vi "Create Plot Object.vi"(6 "Control Ref Queue":T1, 7 "Actual Transform In":T2, 8 "error in (no error)":errorcluster, 9 "Multiplot Representation In":T4, 10 "3D Mesh.lvclass in":refnum<class "3D Waterfall.lvclass">, 11 "Plot Object In":refnum<vi>) -> (0 "error out":errorcluster, 1 "Multiplot Representation Out":T4, 2 "3D Mesh.lvclass out":refnum<class "3D Waterfall.lvclass">, 3 "Plot Object Out":refnum<vi>, 5 "Actual Transform Out":T2)   [LabVIEW 2017, in "3D Waterfall.lvclass"]
uses:
  <vilib>/Math Plots/3D Math Plots/3D Waterfall/3D Waterfall/3D Waterfall.lvclass
  <vilib>/Math Plots/3D Math Plots/3D Plot/3D Plot/Typedef/Multiplot Representation.ctl
  <vilib>/Math Plots/3D Math Plots/3D Plot/3D Plot/Typedef/Plot Representation.ctl
  <vilib>/Math Plots/3D Math Plots/3D Plot/3D Plot/Typedef/Range Clusters.ctl
  <vilib>/Math Plots/3D Math Plots/3D Plot/3D Plot/Typedef/Mesh Data.ctl
  <vilib>/Math Plots/3D Math Plots/3D Plot/3D Plot/Typedef/Actual Transform.ctl
  <vilib>/Math Plots/3D Math Plots/3D Plot/Action String/3DMathPlot Ctrl Act Queue.ctl
  <vilib>/Math Plots/3D Math Plots/3D Plot/Action String/3DMathPlot Ctrl Act Cluster.ctl
  <vilib>/Math Plots/3D Math Plots/3D Plot/Action String/3DMathPlot State Class.ctl
  <vilib>/Math Plots/3D Math Plots/3D Waterfall/3D Waterfall/3D Waterfall.lvclass/3D Waterfall.ctl
  <vilib>/Math Plots/3D Math Plots/3D Plot/3D Plot/3D Plot.lvclass
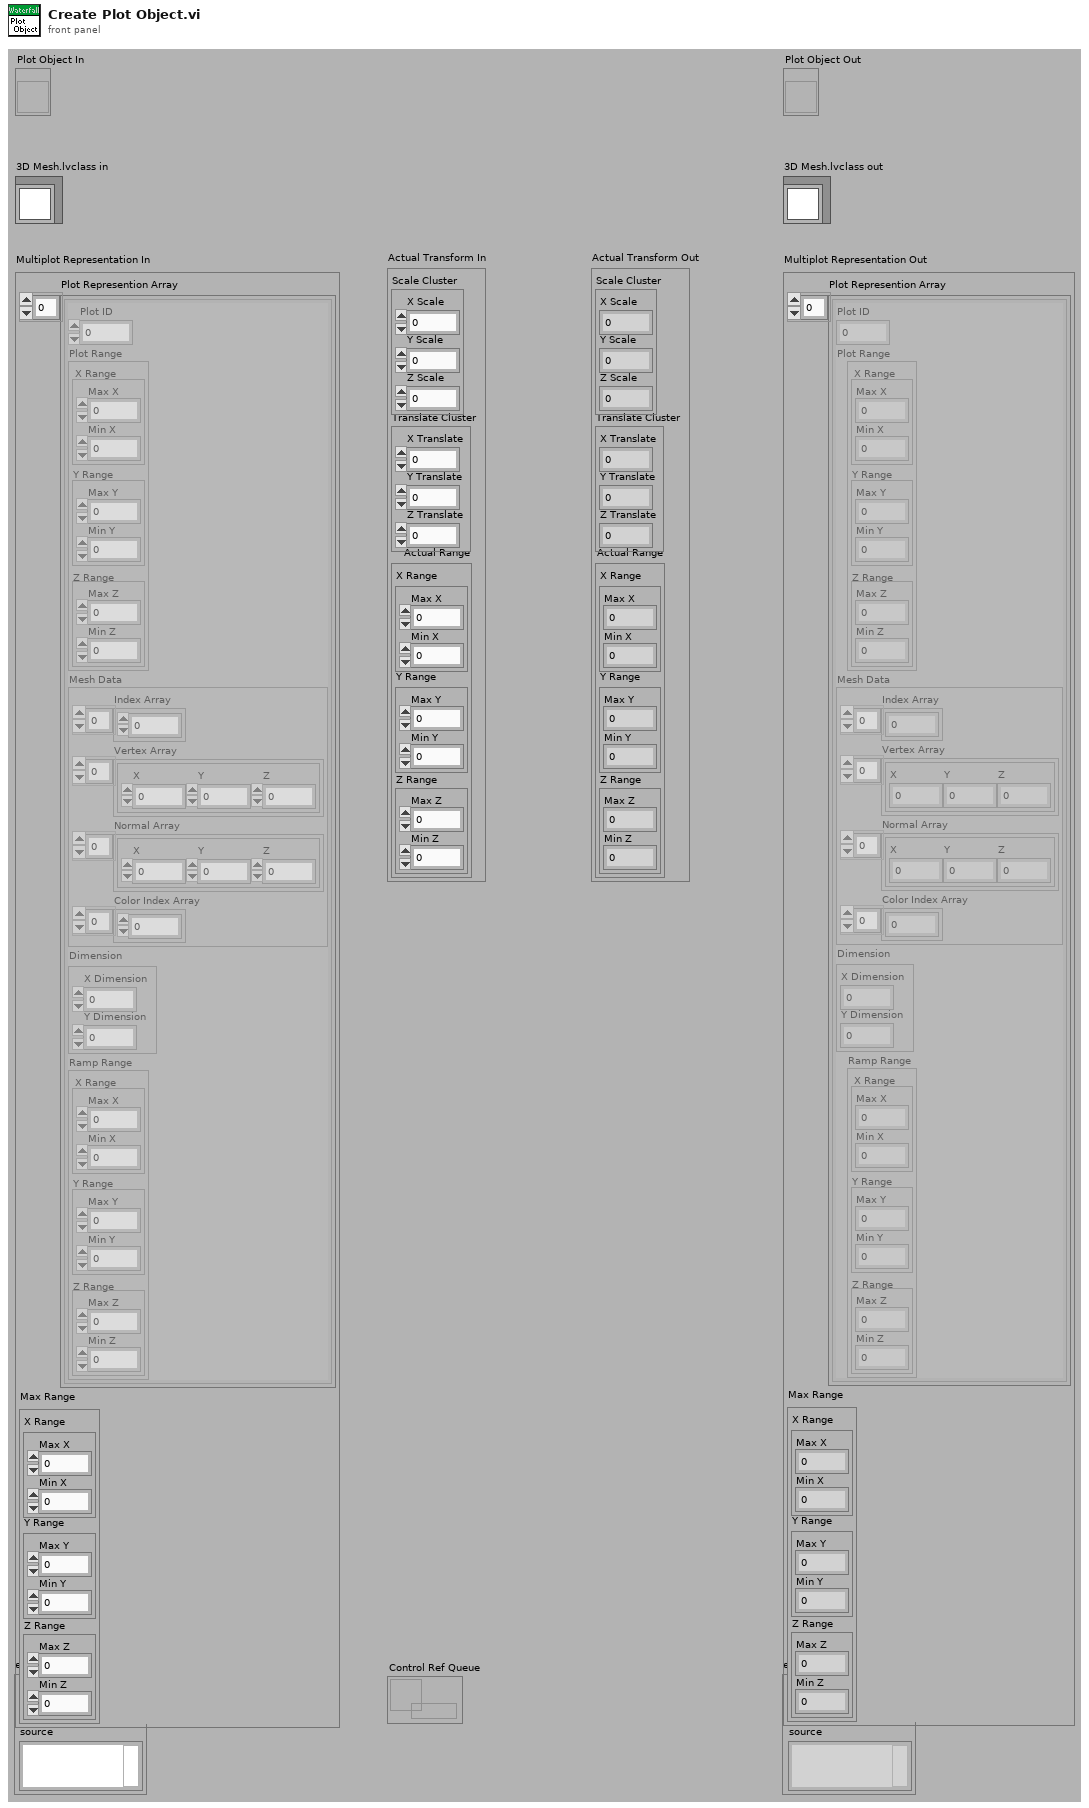
[diagram p1: front panel]
types:
  T1 = typedef "3DMathPlot Ctrl Act Queue.ctl" = refnum<queue>
  T2 = typedef "3D Plot.lvclass/Actual Transform.ctl" = cluster{"Scale Cluster":cluster{"X Scale":sgl, "Y Scale":sgl, "Z Scale":sgl}, "Translate Cluster":cluster{"X Translate":sgl, "Y Translate":sgl, "Z Translate":sgl}, "Actual Range":T3}
  T3 = typedef "3D Plot.lvclass/Range Clusters.ctl" = cluster{"X Range":cluster{"Max X":sgl, "Min X":sgl}, "Y Range":cluster{"Max Y":sgl, "Min Y":sgl}, "Z Range":cluster{"Max Z":sgl, "Min Z":sgl}}
  T4 = typedef "3D Plot.lvclass/Multiplot Representation.ctl" = cluster{"Plot Represention Array":T5[], "Max Range":T3}
  T5 = typedef "3D Plot.lvclass/Plot Representation.ctl" = cluster{"Plot ID":i32, "Plot Range":T3, "Mesh Data":T6, "Dimension":cluster{"X Dimension":i32, "Y Dimension":i32}, "Ramp Range":T3}
  T6 = typedef "3D Plot.lvclass/Mesh Data.ctl" = cluster{"Index Array":u32[], "Vertex Array":cluster{"X":sgl, "Y":sgl, "Z":sgl}[], "Normal Array":cluster{"X":sgl, "Y":sgl, "Z":sgl}[], "Color Index Array":i32[]}
  T7 = typedef "3D Waterfall.lvclass/3D Waterfall Propery Array.ctl" = T8[]
  T8 = typedef "3D Waterfall.lvclass/3D Waterfall Property.ctl" = cluster{"General Property":cluster{"Plot Name":string, "Coordinate System":enum16{"Cartesian", "Cylindrical", "Spherical"}, "Opacity":sgl}, "Projection Property":cluster{"Draw XY":bool, "Draw YZ":bool, "Draw XZ":bool}, "Plot Property":cluster{"Line Style":T9, "Line Width":sgl, "Color Ramp Cluster":T10, "Antialiasing":bool}, "Waterfall Property":cluster{"Waterfall Mode":enum16{"Lines", "Slices"}}}
  T9 = typedef "3D Plot.lvclass/Line Type.ctl" = enum16{"None", "Solid", "Dash", "Dot", "Dash Dot"}
  T10 = typedef "3D Plot.lvclass/Color Ramp Cluster.ctl" = cluster{"Color Ramp Style":enum16{"None", "Shaded", "Color spectrum", "Grey scale", "Custom"}, "Color Ramp Array":u32[], "Color Ramp Index":i32[], "Interpolate?":bool, "Logarithm?":bool}
  T11 = enum16{"Points", "Lines", "Line Strip", "Line Loop", "Triangles", "Triangle Strip", "Triangle Fan", "Quads", "Quad Strip", "Polygon"}
  T12 = cluster{"Draw XY":bool, "Draw YZ":bool, "Draw XZ":bool}
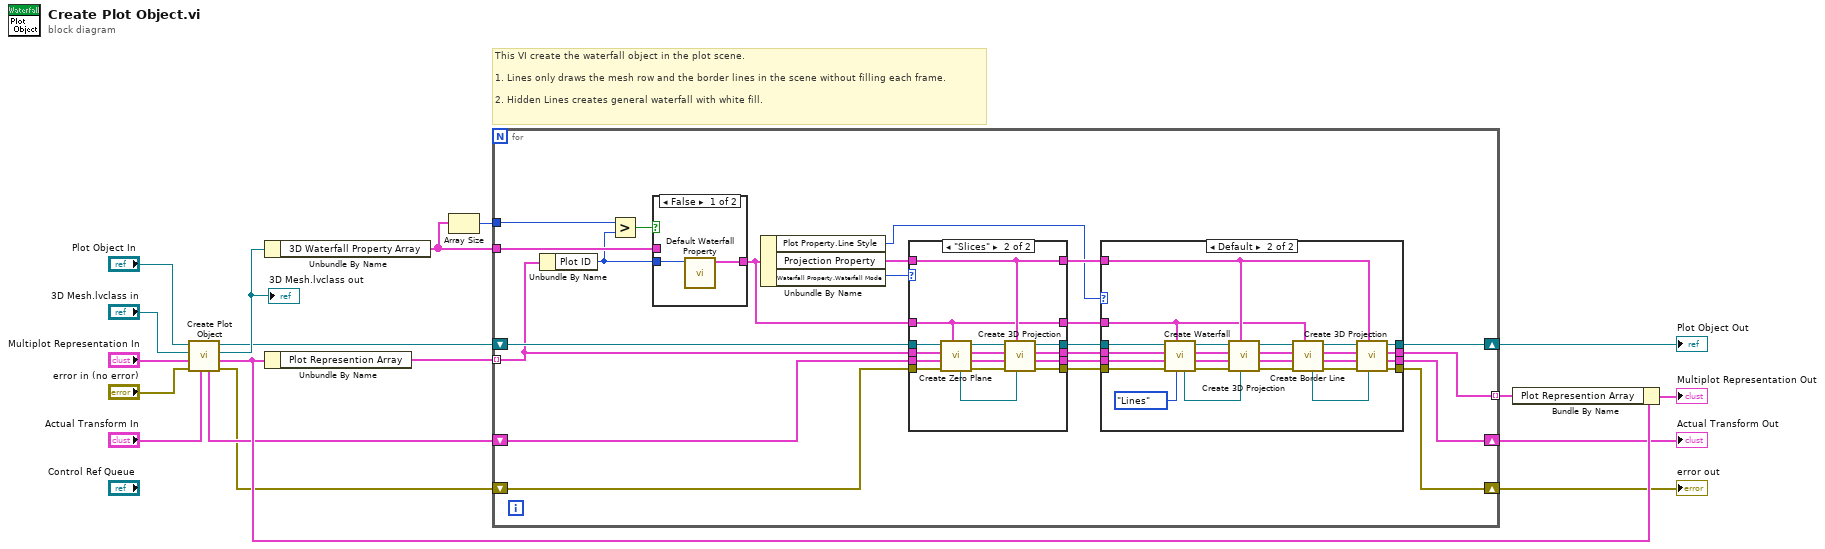
[diagram p0: block diagram]
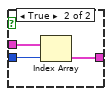
[diagram p2: hidden frame]
diagram:
  # "This VI create the waterfall object in the plot scene.\n\n1. Lines only draws the mesh row and the border lines in the scene without filling each frame.\n\n2. Hidden Lines creates general waterfall with white fill."
  n1 = call-parent "Create Plot Object.vi"("Actual Transform In"="Actual Transform In", "error in (no error)"="error in (no error)", "Multiplot Representation In"="Multiplot Representation In", "3D Plot.lvclass in"="3D Mesh.lvclass in", "Plot Object In"="Plot Object In") -> ("error out"=w5:errorcluster, "Multiplot Representation Out"=w12:T4, "3D Plot.lvclass out"=w6:refnum<class "3D Waterfall.lvclass">, "Plot Object Out"=w4:refnum<vi>, "Actual Transform Out"=w9:T2)  [unwired: 1 in, 1 out]
  "3D Mesh.lvclass out" <- w6
  n2 = Unbundle By Name(w6) -> ("3D Waterfall Property Array"=w2:T7)
  n3 = Unbundle By Name(w12) -> ("Plot Represention Array"=w18:T5[])
  n4 = Array Size(array=w2) -> (size(s)=w1:i32)
  n5 = for {
    shift-right: [w37] -> w7
    shift-left: w5 -> [w33]
    shift-right: [w40] -> w3
    shift-left: w4 -> [w36]
    shift-right: [w38] -> w8
    shift-left: w9 -> [w34]
    tunnel: w18 -> [w35] mode=indexing
    tunnel: [w39] -> w17 mode=indexing
    tunnel: w2 -> [w21]
    tunnel: w1 -> [w22]
    n6 = Unbundle By Name(w35) -> ("Plot ID"=w19:i32)
    n7 = Greater?(x=w22, y=w19) -> (0:w23:bool)
    n8 = case shown="False" w23 {
      tunnel: w21 -> [_ w45]
      tunnel: [w41 w44] -> w20
      tunnel: w19 -> [w42 w43]
      frame False {
        n9 = call <vilib>:"Default Waterfall Property.vi"("Plot ID"=w42) -> ("Default Property"=w41:T8)  [unwired: 10 out]
      }
      frame True {
        n10 = Index Array(array=w45, index=w43) -> (element=w44:T8)
      }
    }
    n11 = Unbundle By Name(w20) -> ("Plot Property.Line Style"=w24:T9, "Projection Property"=w32:T12, "Waterfall Property.Waterfall Mode"=w25:enum16{"Lines", "Slices"})
    n12 = case shown="\"Slices\"" w25 {
      tunnel: [w78 w92] -> w30
      tunnel: [w76 w91] -> w29
      tunnel: [w77 w90] -> w28
      tunnel: [w75 w89] -> w27
      tunnel: w32 -> [w74 w80]
      tunnel: w33 -> [w75 w84]
      tunnel: w34 -> [w76 w83]
      tunnel: w36 -> [w78 w82]
      tunnel: w35 -> [w77 w81]
      tunnel: w20 -> [w73 w79]
      tunnel: [w74 w80] -> w31
      tunnel: [w73 w79] -> w26
      frame "Lines", Default {
      }
      frame "Slices" {
        n13 = call <vilib>:"Create Zero Plane.vi"("3D Waterfall Property"=w79, "error in (no error)"=w84, "Actual Transform In"=w83, "Plot Representation In"=w81, "Plot Object In"=w82) -> ("error out"=w88:errorcluster, "Actual Transform Out"=w86:T2, "Plot Representation Out"=w90:T5, "Plot Object Out"=w87:refnum<vi>, "Zero Plane Object Out"=w85:refnum<vi>)  [unwired: 1 in, 1 out]
        n14 = call <vilib>:"Create 3D Projection.vi"("Sub Object In"=w85, "Projection Property"=w80, "error in (no error)"=w88, "Actual Transform In"=w86, "Plot Object In"=w87) -> ("error out"=w89:errorcluster, "Actual Transform Out"=w91:T2, "Plot Object Out"=w92:refnum<vi>)  [unwired: 1 in, 3 out]
      }
    }
    n15 = case shown="Default" w24 {
      tunnel: [w49 w60] -> w40
      tunnel: [w48 w59] -> w39
      tunnel: [w47 w58] -> w38
      tunnel: [w46 w57] -> w37
      tunnel: w31 -> [_ w56]
      tunnel: w30 -> [w49 w55]
      tunnel: w29 -> [w47 w54]
      tunnel: w28 -> [w48 w53]
      tunnel: w27 -> [w46 w52]
      tunnel: w26 -> [_ w50]
      frame "None" {
      }
      frame Default {
        n16 = call <vilib>:"Create Waterfall.vi"("Draw Mode"=T11."Lines", "3D Waterfall Property"=w50, "error in (no error)"=w52, "Actual Transform In"=w54, "Plot Representation In"=w53, "Plot Object In"=w55) -> ("error out"=w72:errorcluster, "Actual Transform Out"=w71:T2, "Plot Representation Out"=w65:T5, "Plot Object Out"=w70:refnum<vi>, "Waterfall Object Out"=w69:refnum<vi>)  [unwired: 1 in]
        n17 = call <vilib>:"Create 3D Projection.vi"("Sub Object In"=w69, "Projection Property"=w56, "error in (no error)"=w72, "Actual Transform In"=w71, "Plot Object In"=w70) -> ("error out"=w66:errorcluster, "Actual Transform Out"=w67:T2, "Plot Object Out"=w68:refnum<vi>)  [unwired: 1 in, 3 out]
        n18 = call <vilib>:"Create Border Line.vi"("3D Waterfall Property"=w50, "error in (no error)"=w66, "Actual Transform In"=w67, "Plot Representation In"=w65, "Plot Object In"=w68) -> ("error out"=w63:errorcluster, "Actual Transform Out"=w62:T2, "Plot Representation Out"=w59:T5, "Plot Object Out"=w61:refnum<vi>, "Border Line Object Out"=w64:refnum<vi>)  [unwired: 1 in, 1 out]
        n19 = call <vilib>:"Create 3D Projection.vi"("Sub Object In"=w64, "Projection Property"=w56, "error in (no error)"=w63, "Actual Transform In"=w62, "Plot Object In"=w61) -> ("error out"=w57:errorcluster, "Actual Transform Out"=w58:T2, "Plot Object Out"=w60:refnum<vi>)  [unwired: 1 in, 3 out]
      }
    }
  }
  "error out" <- w7
  "Plot Object Out" <- w3
  "Actual Transform Out" <- w8
  n20 = Bundle By Name(cluster=w12, "Plot Represention Array"=w17) -> (→"Multiplot Representation Out":T4)
